vi "Read Date and Time.vi"(8 "error in (no error)":errorcluster, 11 "VGC in":refnum<class "PL Inficon VGC.lvclass">) -> (0 "error out":errorcluster, 2 "date and time":timestamp, 3 "VGC out":refnum<class "PL Inficon VGC.lvclass">)   [LabVIEW 2015, in "PL Inficon VGC.lvclass"]
doc: "Reads date and time."
uses:
  PL Inficon VGC.lvclass
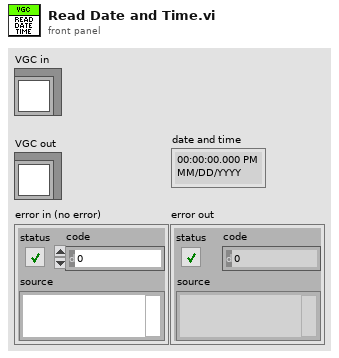
[diagram p1: front panel]
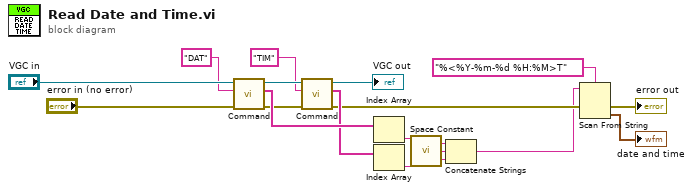
[diagram p0: block diagram]
diagram:
  n1 = call "Command.vi"("error in (no error)"="error in (no error)", "command"="DAT" ("format string"), "VGC in"="VGC in") -> ("error out"=w9:errorcluster, "response data"=w12:string[], "VGC out"=w11:refnum<class "PL Inficon VGC.lvclass">)  [unwired: 6 in]
  n2 = call "Command.vi"("error in (no error)"=w9, "command"="TIM" ("format string"), "VGC in"=w11) -> ("error out"=w3:errorcluster, "response data"=w7:string[], "VGC out"=→"VGC out":refnum<class "PL Inficon VGC.lvclass">)  [unwired: 6 in]
  n3 = Index Array(array=w12) -> (element=w6:string)  [unwired: 1 in]
  n4 = Index Array(array=w7) -> (element=w5:string)  [unwired: 1 in]
  n5 = call <vilib>:"Space Constant.vi"() -> ("String"=w13:string)
  n6 = Concatenate Strings(w6, w13, w5) -> (w1:string)
  n7 = Scan From String(format string="%<%Y-%m-%d %H:%M>T", input string=w1, error in=w3) -> (error out=→"error out":errorcluster, output 1=→"date and time":timestamp)  [unwired: 2 in, 2 out]
